vi "unpack tcp packet.vi"(11 "TCP Pack":string="\u0000resp      啊手动阀手动阀") -> (2 "tcp-message-type":T1=enum."resp", 3 "String":string="啊手动阀手动阀")   [LabVIEW 2020, in "CSM-TCP-Router.lvlib"]
uses:
  CSM-TCP-Router.lvlib
  tcp-msg type.ctl
  <userlib>/_NEVSTOP/Communicable State Machine(CSM)/addons/MassData-Parameter/_support/Operation-FGV-MassData.ctl
  <userlib>/_NEVSTOP/Communicable State Machine(CSM)/addons/MassData-Parameter/CSM MassData Parameter Support.lvlib
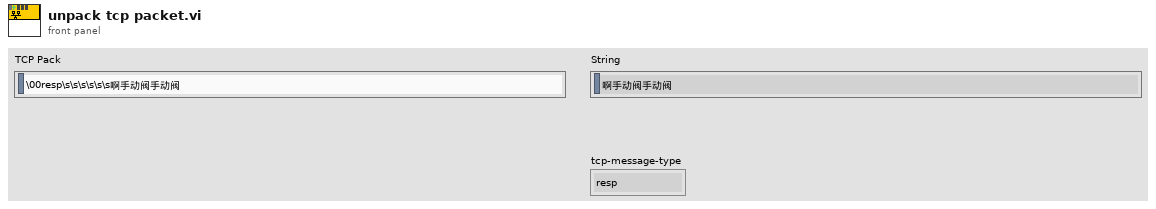
[diagram p1: front panel]
types:
  T1 = typedef "CSM-TCP-Router.lvlib/tcp-msg type.ctl" = enum8{"info", "error", "cmd", "cmd-resp", "resp", "async-resp", "status", "interrupt"}
  T2 = typedef "CSM MassData Parameter Support.lvlib/Operation-FGV-MassData.ctl" = enum16{"Initialize", "Read", "Write", "Status", "Release"}
  T3 = typedef "CSM MassData Parameter Support.lvlib/Def-MassDataOper-Status.ctl" = cluster{"Start":i32, "Size":i32, "Total":i32}
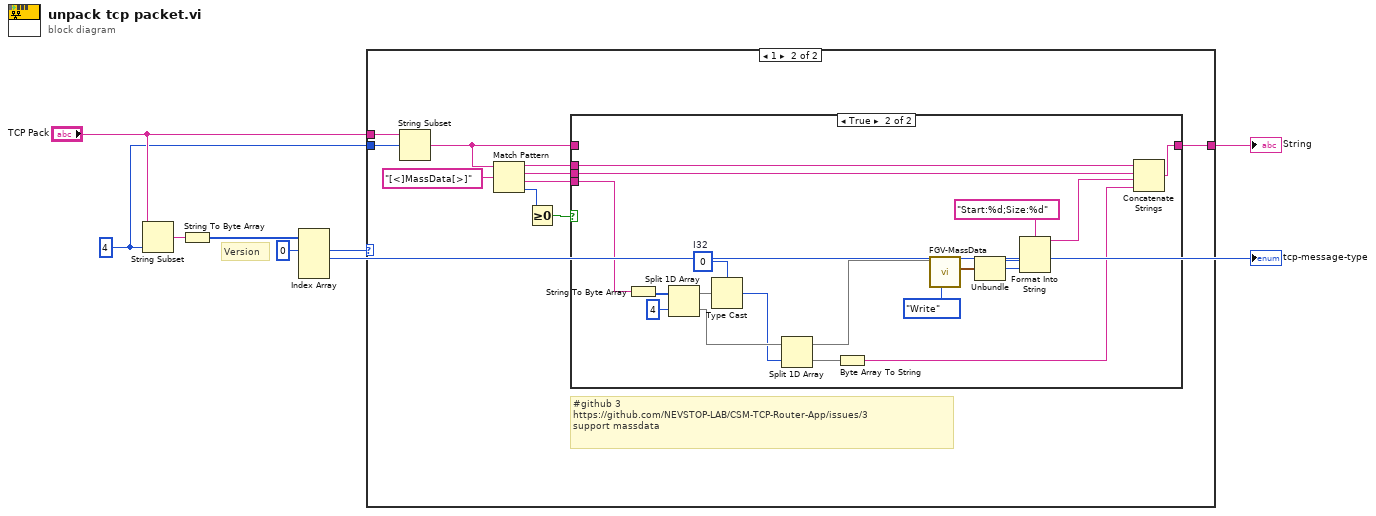
[diagram p0: block diagram]
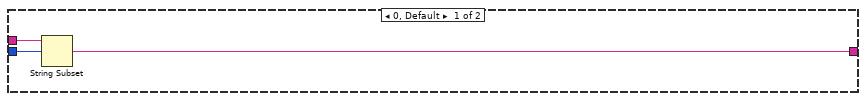
[diagram p2: hidden frame]
diagram:
  w3 = 4 ("length (rest)")
  # "Version"
  n1 = String Subset(string="TCP Pack", length (rest)=w3) -> (substring=w8:string)  [unwired: 1 in]
  n2 = String To Byte Array(string=w8) -> (unsigned byte array=w7:u8[])
  n3 = Index Array(array=w7, index #1=0 ("index")) -> (element #1=w1:u8, element #2=→"tcp-message-type":u8)  [unwired: 3 in, 2 out]
  n4 = case shown="1" w1 {
    tunnel: "TCP Pack" -> [w11 w21]
    tunnel: [w10 w12] -> w5
    tunnel: w3 -> [w9 w20]
    frame 0, Default {
      n5 = String Subset(string=w11, offset (0)=w9) -> (substring=w10:string)  [unwired: 1 in]
    }
    frame 1 {
      # "#github 3\nhttps://github.com/NEVSTOP-LAB/CSM-TCP-Router-App/issues/3\nsupport massdata"
      n6 = String Subset(string=w21, offset (0)=w20) -> (substring=w13:string)  [unwired: 1 in]
      n7 = Match Pattern(string=w13, regular expression="[<]MassData[>]" ("string")) -> (before substring=w17:string, match substring=w16:string, after substring=w15:string, offset past match=w18:i32)  [unwired: 1 in]
      n8 = Greater Or Equal To 0?(x=w18) -> (x >= 0?=w14:bool)
      n9 = case shown="True" w14 {
        tunnel: w17 -> [_ w41]
        tunnel: w16 -> [_ w40]
        tunnel: w15 -> [_ w39]
        tunnel: [w22 w23] -> w12
        tunnel: w13 -> [w22 _]
        frame False {
        }
        frame True {
          w35 = 0  # I32
          n10 = String To Byte Array(string=w39) -> (unsigned byte array=w38:u8[])
          n11 = Split 1D Array(array=w38, index=4) -> (first subarray=w36:u8[], second subarray=w34:u8[])
          n12 = Type Cast(type=w35, x=w36) -> (*(type *) &x=w33:i32)
          n13 = Split 1D Array(array=w34, index=w33) -> (first subarray=w25:u8[], second subarray=w32:u8[])
          n14 = Byte Array To String(unsigned byte array=w32) -> (string=w31:string)
          n15 = call <userlib>:"FGV-MassData.vi"("Operation"=Operation-FGV-MassData."Write", "Data in"=w25) -> ("Active Write Oper"=w29:T3)  [unwired: 6 in, 3 out]
          n16 = Unbundle(w29) -> ("Start"=w28:i32, "Size"=w27:i32)  [unwired: 1 out]
          n17 = Format Into String(format string="Start:%d;Size:%d", w28, w27) -> (resulting string=w24:string)  [unwired: 2 in, 1 out]
          n18 = Concatenate Strings(w41, w40, w24, w31) -> (w23:string)
        }
      }
    }
  }
  "String" <- w5
